vi "Initialize Modbus Master Connection.vi"(8 "error in (no error)":errorcluster, 11 "Parameters":T1={"Interface Data"={"Name"="", "Unit ID"=0, "Refresh Rate"=0, "Write Rate"=0, "Write Mode"=enum."Value Change", "Interface Type"=enum."TCP Master", "TCP Settings"={"Address"="", "Port"=0, "Timeout"=0}, "Serial Settings"={"VISA resource name"="", "baud rate"=0, "parity (even)"=0, "flow control (none)"=0, "serial type"=enum."RTU", "Wire Mode"=-1}}, "Modbus Input Groups"=[], "Modbus Output Groups"=[], "error in (no error)"={"status"=FALSE, "code"=0, "source"=""}, "Modbus Input Engine Group Names"=[], "Modbus Output Engine Group Names"=[]} {"Interface Data"."Serial Settings"."Wire Mode" items=["Unknown"=-1, "RS485/Wire4"=0, "RS485/Wire2-EchoDTR"=1, "RS485/Wire2-CtrlDTR"=2, "RS485/Wire2-Auto"=3, "RS232/DTE"=128, "RS232/DCE"=129, "RS232/AUTO"=130]; "Interface Data"."Serial Settings"."parity (even)" items=["None", "Odd", "Even", "Mark", "Space"]; "Interface Data"."Serial Settings"."flow control (none)" items=["None", "XON/XOFF", "RTS/CTS", "XON/XOFF & RTS/CTS", "DTR/DSR", "XON/XOFF & DTR/DSR"]}) -> (0 "error out":errorcluster, 3 "Modbus Master out":refnum<class "Modbus Master.lvclass">)   [LabVIEW 2020, in "Modbus Master Engine.lvlib"]
uses:
  Modbus Master Engine.lvlib
  Custom Device/Shared/Device Info.ctl
  Custom Device/Shared/Write Mode.ctl
  Custom Device/Shared/Controls/Interface Type.ctl
  Custom Device/Shared/Controls/Data Model/TCP Settings.ctl
  Custom Device/Shared/Controls/Data Model/Serial Settings.ctl
  Custom Device/Shared/Bulk Data Access.ctl
  Custom Device/System Explorer/SubVIs/Modbus Type.ctl
  Custom Device/Shared/Controls/Data Model/Channel.ctl
  <vilib>/NI VeriStand/Custom Device API/Custom Device Channel Type.ctl
  Custom Device/Shared/Controls/Data Model/Mapping.ctl
  Custom Device/Shared/Controls/Data Model/DataType.ctl
  <vilib>/NI VeriStand/Custom Device API/Custom Device Item Ref.ctl
  API/Master/Modbus Master.lvclass
  C:/Users/Administrator/Desktop/GIT/Modbus-Custom-Device-v2/Source/Custom Device Support/API/Modbus API.lvclass
  API/Modbus API.lvclass/Modbus API.ctl
  Transmission Data Unit/Transmission Data Unit.lvclass/Transmission Data Unit.ctl
  API/Master/Set Read Timeout.vi
  API/Master/Set Write Timeout.vi
  API/Read Transmission Data Unit.vi
  API/Write Transmission Data Unit.vi
  Transmission Data Unit/Write read operation timeout.vi
  Transmission Data Unit/Write write operation timeout.vi
  API/Wrapper/API Main.lvlib
  <vilib>/NI VeriStand/Custom Device Tools/Custom Device Utility Library/Custom Device Utility Library.lvlib
  Custom Device/Shared/Modbus Master Shared.lvlib
  <vilib>/NI VeriStand/Custom Device API/Custom Device API.lvlib
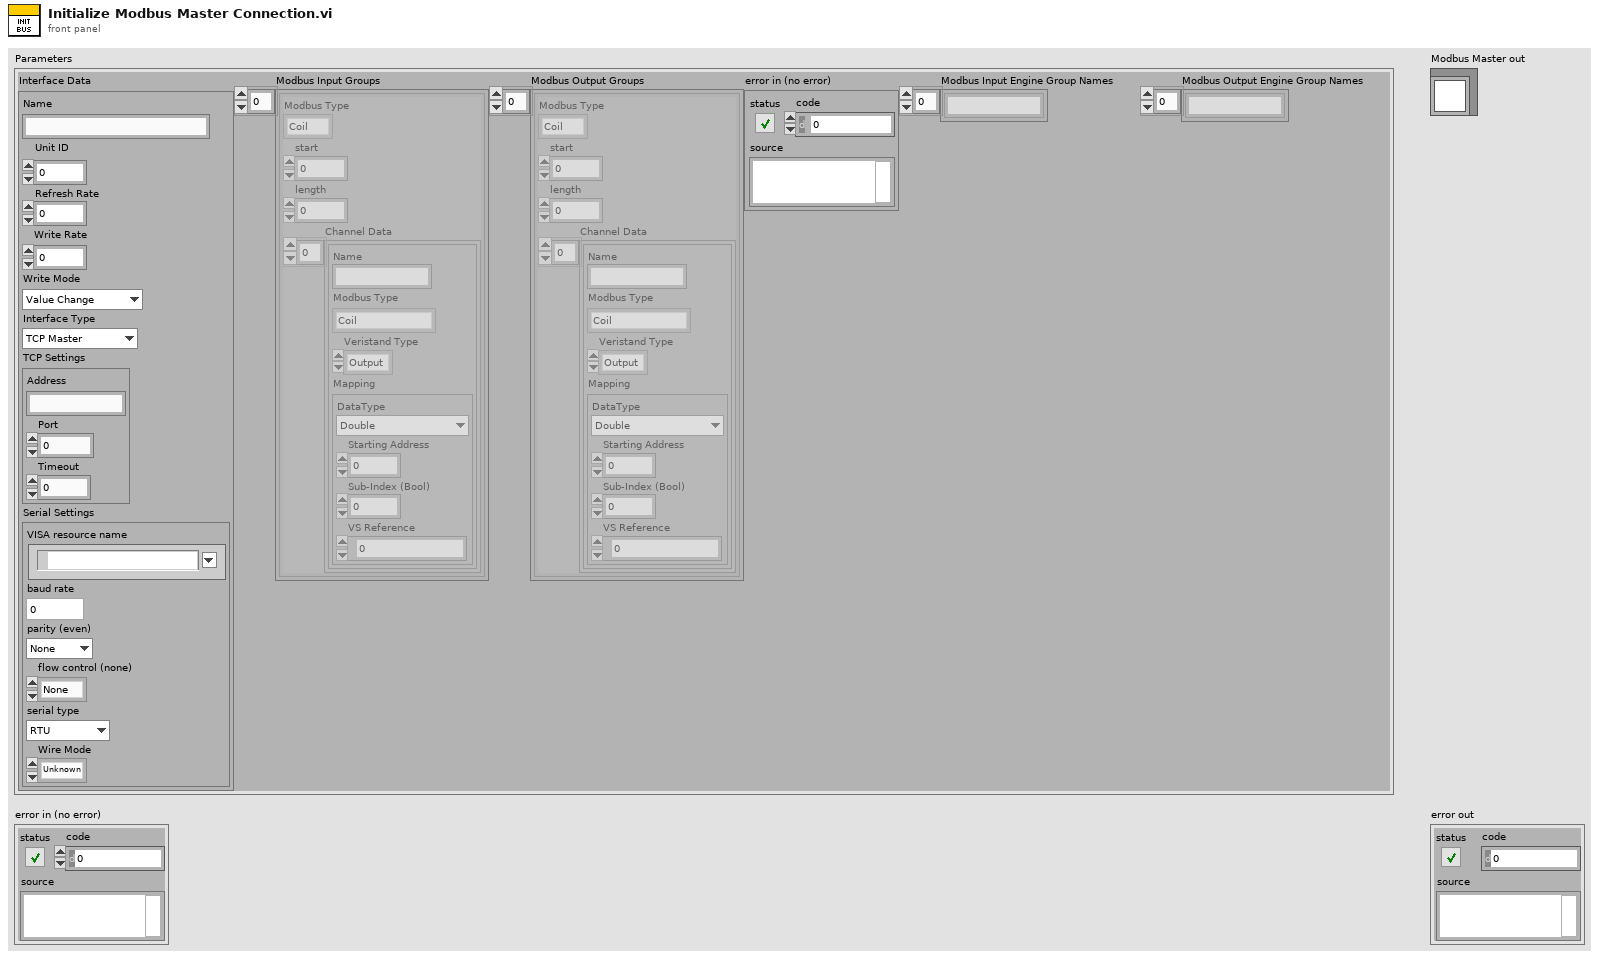
[diagram p1: front panel]
types:
  T1 = typedef "Modbus Master Shared.lvlib/Device Info.ctl" = cluster{"Interface Data":cluster{"Name":string, "Unit ID":u8, "Refresh Rate":i32, "Write Rate":i32, "Write Mode":T2, "Interface Type":T3, "TCP Settings":T4, "Serial Settings":T5}, "Modbus Input Groups":T6[], "Modbus Output Groups":T6[], "error in (no error)":errorcluster, "Modbus Input Engine Group Names":string[], "Modbus Output Engine Group Names":string[]}
  T2 = typedef "Modbus Master Shared.lvlib/Write Mode.ctl" = enum16{"Value Change", "Interval"}
  T3 = typedef "Modbus Master Shared.lvlib/Interface Type.ctl" = enum16{"TCP Master", "Serial Master", "TCP Slave", "Serial Slave"}
  T4 = typedef "Modbus Master Shared.lvlib/TCP Settings.ctl" = cluster{"Address":string, "Port":u16, "Timeout":i32}
  T5 = typedef "Modbus Master Shared.lvlib/Serial Settings.ctl" = cluster{"VISA resource name":refnum<visa-resource-name>, "baud rate":u32, "parity (even)":u16, "flow control (none)":u16, "serial type":enum16{"RTU", "ASCII"}, "Wire Mode":i16}
  T6 = typedef "Modbus Master Shared.lvlib/Bulk Data Access.ctl" = cluster{"Modbus Type":T7, "start":u16, "length":u16, "Channel Data":T8[]}
  T7 = typedef "Modbus Master Shared.lvlib/Modbus Type.ctl" = enum16{"Coil", "Discrete Input", "Holding Register", "Input Register"}
  T8 = typedef "Modbus Master Shared.lvlib/Channel.ctl" = cluster{"Name":string, "Modbus Type":T7, "Veristand Type":T9, "Mapping":T10}
  T9 = typedef "Custom Device API.lvlib/Custom Device Channel Type.ctl" = enum16{"Input", "Output"}
  T10 = typedef "Modbus Master Shared.lvlib/Mapping.ctl" = cluster{"DataType":T11, "Starting Address":u16, "Sub-Index (Bool)":u16, "VS Reference":T12}
  T11 = typedef "Modbus Master Shared.lvlib/DataType.ctl" = enum16{"Double", "Single", "I64", "I32", "I16", "I8", "U64", "U32", "U16", "U8", "Boolean"}
  T12 = typedef "Custom Device API.lvlib/Custom Device Item Ref.ctl" = u64
  T13 = cluster{"serial master instances":refnum<class "Modbus Master.lvclass">[], "VISA Resources":refnum<visa-resource-name>[]}
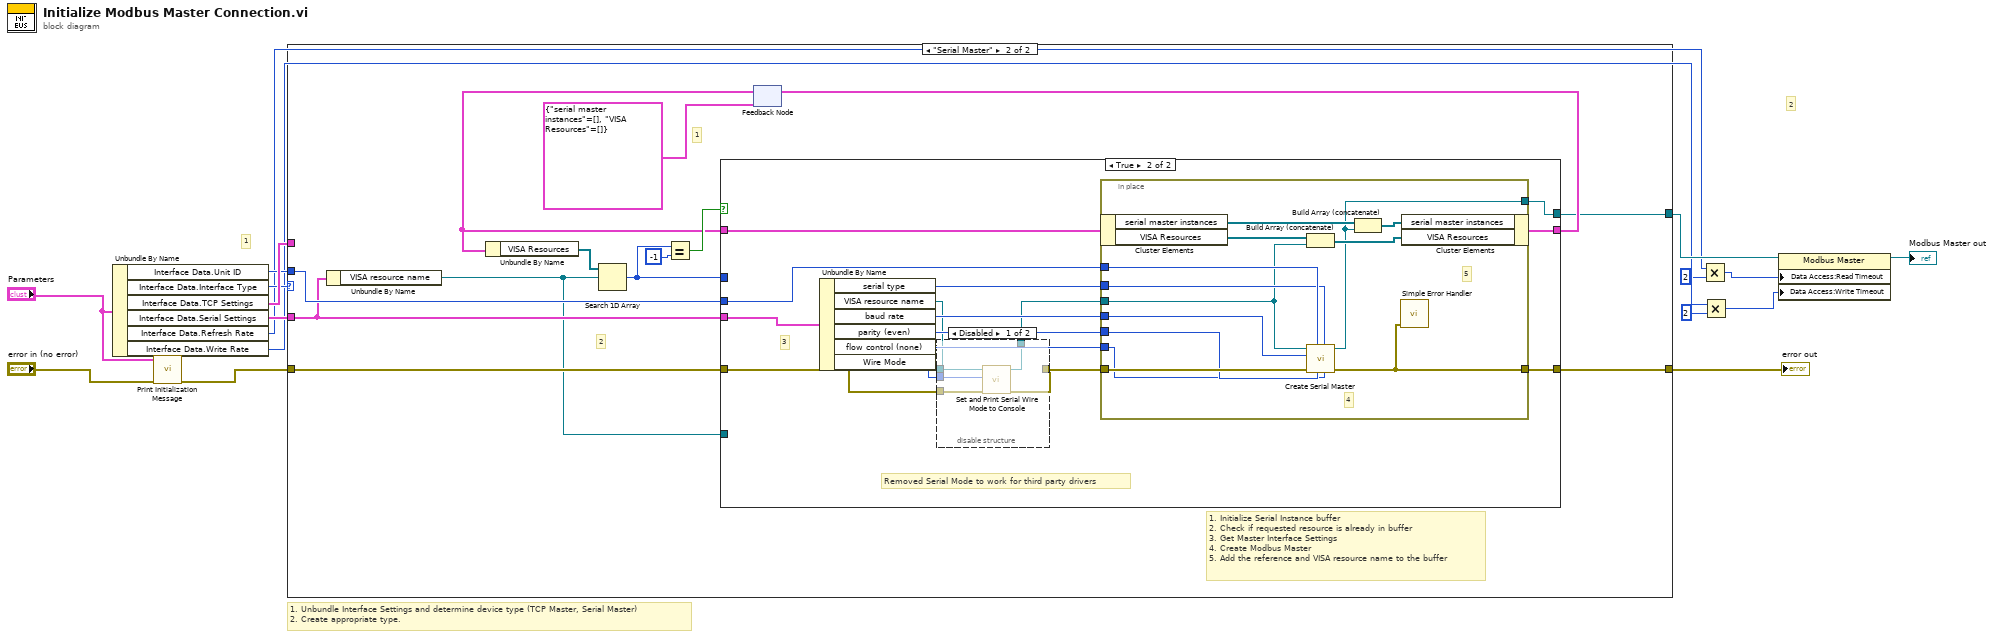
[diagram p0: block diagram]
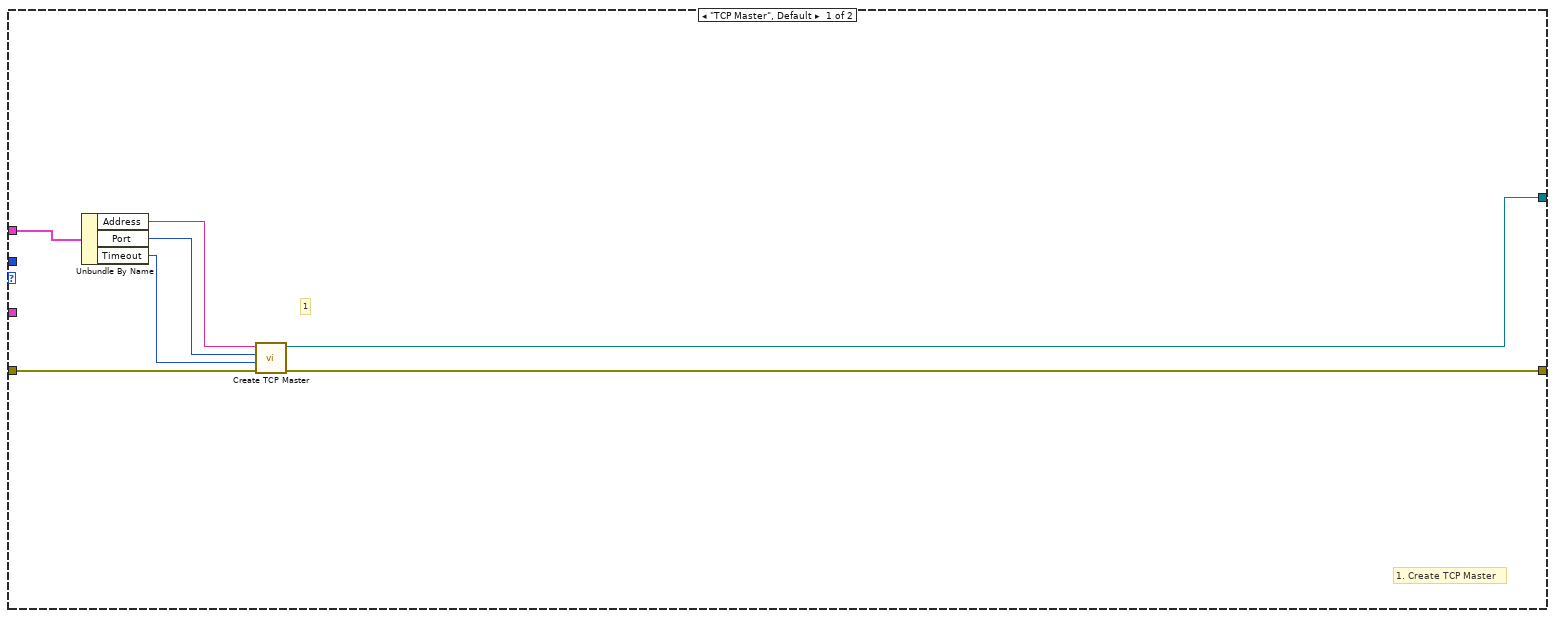
[diagram p2: hidden frame]
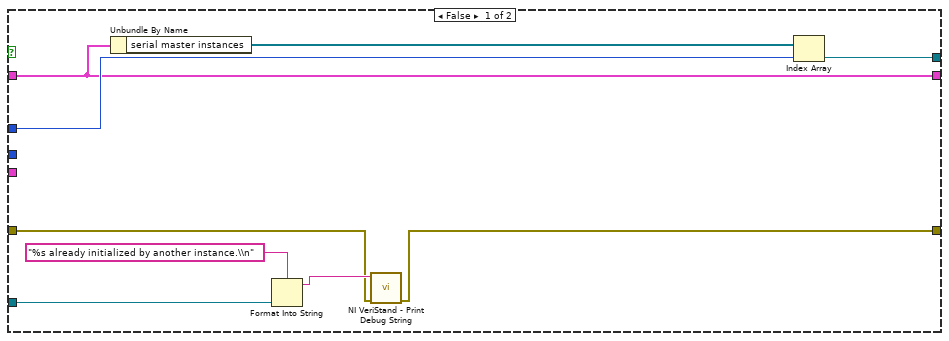
[diagram p3: hidden frame]
diagram:
  # "2"
  # "1"
  # "1. Unbundle Interface Settings and determine device type (TCP Master, Serial Master)\n2. Create appropriate type."
  n1 = Unbundle By Name("Parameters") -> ("Interface Data.Unit ID"=w13:u8, "Interface Data.Interface Type"=w14:T3, "Interface Data.TCP Settings"=w15:T4, "Interface Data.Serial Settings"=w16:T5, "Interface Data.Refresh Rate"=w6:i32, "Interface Data.Write Rate"=w5:i32)
  n2 = call "Print Initialization Message.vi"("error in (no error)"="error in (no error)", "Parameters"="Parameters") -> ("error out"=w10:errorcluster)  [unwired: 9 in]
  n3 = case shown="\"Serial Master\"" w14 {
    tunnel: w13 -> [_ w36]
    tunnel: w15 -> [w23 _]
    tunnel: w16 -> [_ w31]
    tunnel: [w20 w25] -> w8
    tunnel: [w19 w29] -> w9
    tunnel: w10 -> [w18 w30]
    frame "TCP Master", Default {
      # "1. Create TCP Master"
      # "1"
      n4 = Unbundle By Name(w23) -> ("Address"=w22:string, "Port"=w21:u16, "Timeout"=w17:i32)
      n5 = call "Create TCP Master.vi"("error in"=w18, "connect timeout ms"=w17, "port (502)"=w21, "address"=w22) -> ("error out"=w19:errorcluster, "TCP master instance"=w20:refnum<class "Modbus Master.lvclass">)  [unwired: 6 in]
    }
    frame "Serial Master" {
      # "1. Initialize Serial Instance buffer\n2. Check if requested resource is already in buffer\n3. Get Master Interface Settings\n4. Create Modbus Master\n5. Add the reference and VISA resource name to the buffer"
      # "2"
      # "1"
      n6 = Unbundle By Name(w31) -> ("VISA resource name"=w24:refnum<visa-resource-name>)
      n7 = feedback #1(T13 {"serial master instances"=[], "VISA Resources"=[]}) -> (w27:T13)
      n8 = Unbundle By Name(w27) -> ("VISA Resources"=w26:refnum<visa-resource-name>[])
      n9 = Search 1D Array(1D array=w26, element=w24) -> (index of element=w34:i32)  [unwired: 1 in]
      n10 = Equal?(x=w34, y=-1) -> (x = y?=w28:bool)
      n11 = case shown="True" w28 {
        tunnel: w36 -> [_ w60]
        tunnel: [w37 w59] -> w29
        tunnel: w30 -> [w38 w50]
        tunnel: [w43 w58] -> w25
        tunnel: w34 -> [w45 _]
        tunnel: w27 -> [w42 w57]
        tunnel: [w42 w56] -> w32
        tunnel: w31 -> [_ w55]
        tunnel: w24 -> [w39 _]
        frame False {
          n12 = Unbundle By Name(w42) -> ("serial master instances"=w44:refnum<class "Modbus Master.lvclass">[])
          n13 = Format Into String(format string="%s already initialized by another instance.\\n", w39) -> (resulting string=w41:string)  [unwired: 2 in, 1 out]
          n14 = call <vilib>:"NI VeriStand - Print Debug String.vi"("error in (no error)"=w38, "Message"=w41) -> ("error out"=w37:errorcluster)  [unwired: 9 in]
          n15 = Index Array(array=w44, index=w45) -> (element=w43:refnum<class "Modbus Master.lvclass">)
        }
        frame True {
          # "Removed Serial Mode to work for third party drivers"
          # "3"
          n16 = Unbundle By Name(w55) -> ("serial type"=w54:enum16{"RTU", "ASCII"}, "VISA resource name"=w48:refnum<visa-resource-name>, "baud rate"=w53:u32, "parity (even)"=w52:u16, "flow control (none)"=w51:u16, "Wire Mode"=w46:i16)
          n17 = disable-structure shown="Disabled" {
            disable-tunnel: w50 -> [w65 w66]
            disable-tunnel: [w64 w67] -> w49
            disable-tunnel: w48 -> [w63 w67]
            disable-tunnel: [w62 w66] -> w47
            disable-tunnel: w46 -> [w61 _]
            frame Disabled {
              n18 = call "Set and Print Serial Wire Mode to Console.vi"("error in (no error)"=w65, "Wire Mode"=w61, "VISA Refnum in"=w63) -> ("error out"=w62:errorcluster, "VISA Refnum out"=w64:refnum<visa-resource-name>)  [unwired: 7 in]
            }
            frame Enabled {
            }
          }
          n19 = in-place {
            in-place-border: w60 -> [w80]
            in-place-border: [w68] -> w59
            in-place-border: w47 -> [w79]
            in-place-border: [w70] -> w58
            in-place-border: w54 -> [w74]
            in-place-border: w49 -> [w69]
            in-place-border: w53 -> [w73]
            in-place-border: w52 -> [w72]
            in-place-border: w51 -> [w71]
            # "5"
            # "4"
            n20 = in-place-cluster #2(w57) -> ("serial master instances"=w76:refnum<class "Modbus Master.lvclass">[], "VISA Resources"=w78:refnum<visa-resource-name>[])
            n21 = Build Array (concatenate)(w78, w69) -> (w77:refnum<visa-resource-name>[])
            n22 = call "Create Serial Master.vi"("flow control (none)"=w71, "serial type"=w74, "parity (even)"=w72, "unit ID"=w80, "error in"=w79, "baud rate"=w73, "VISA resource name"=w69) -> ("error out"=w68:errorcluster, "serial master instance"=w70:refnum<class "Modbus Master.lvclass">)  [unwired: 3 in]
            n23 = Build Array (concatenate)(w76, w70) -> (w75:refnum<class "Modbus Master.lvclass">[])
            n24 = call <vilib>:"Simple Error Handler.vi"("error in (no error)"=w68) -> ()  [unwired: 4 in, 5 out]
            n25 = in-place-cluster #2("serial master instances"=w75, "VISA Resources"=w77) -> (w56:T13)
          }
        }
      }
      n26 = feedback-in #1(w32) -> ()
    }
  }
  "error out" <- w9
  n27 = Multiply(x=w6, y=2) -> (x*y=w2:i32)
  n28 = Multiply(x=w5, y=2) -> (x*y=w1:i32)
  n29 = property class="Modbus Master"(reference=w8, "Data Access:Read Timeout"=w2, "Data Access:Write Timeout"=w1) -> (reference out=→"Modbus Master out":refnum<class "Modbus Master.lvclass">)  [unwired: 1 in, 1 out]
